vi "Edit Control File.vi"(0 "Control File Path":path, 5 "Measurement Name":string, 9 "Version":string, 11 "error in (no error)":errorcluster) -> (15 "error out":errorcluster)   [LabVIEW 2021, in "Packager Helpers.lvlib"]
uses:
  Packager Helpers.lvlib
  controls/Config File Operations.ctl
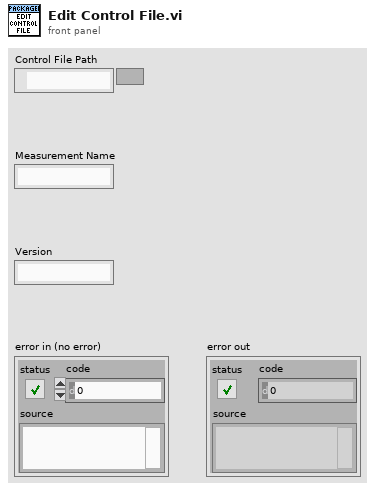
[diagram p1: front panel]
types:
  T1 = typedef "Packager Helpers.lvlib/Config File Operations.ctl" = enum16{"Read", "Write"}
  T2 = enum16{"open", "replace", "create", "open or create", "replace or create", "replace or create with confirmation"}
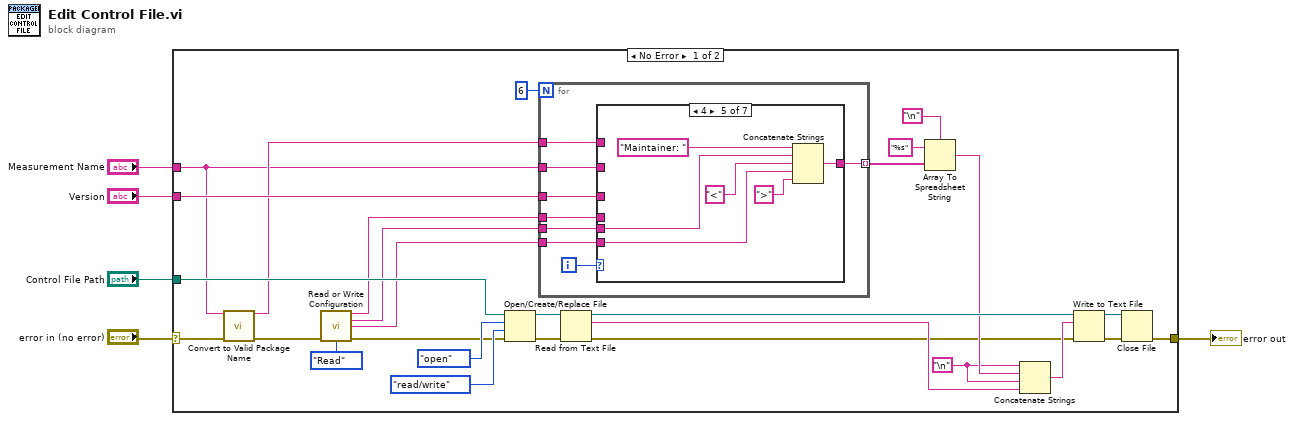
[diagram p0: block diagram]
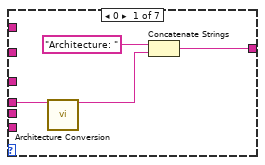
[diagram p2: hidden frame]
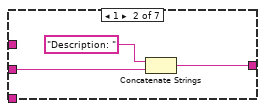
[diagram p3: hidden frame]
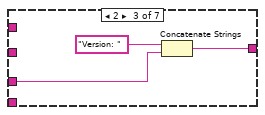
[diagram p4: hidden frame]
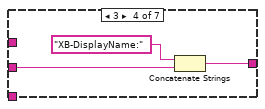
[diagram p5: hidden frame]
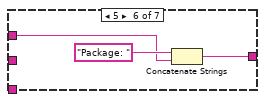
[diagram p6: hidden frame]
diagram:
  n1 = case shown="No Error" "error in (no error)" {
    selector: "error in (no error)" -> [w11 w64]
    tunnel: "Control File Path" -> [w33 _]
    tunnel: [w12 w64] -> w1
    tunnel: "Measurement Name" -> [w6 _]
    tunnel: "Version" -> [w17 _]
    frame No Error {
      w7 = "\n"
      n2 = call "Convert to Valid Package Name.vi"("Package Name"=w6, "error in (no error)"=w11) -> ("Valid Package Name"=w16:string, "error out"=w8:errorcluster)  [unwired: 12 in]
      n3 = call "Read or Write Configuration.vi"("error in (no error)"=w8, "Operation"=Config_File_Operations."Read") -> ("Architecture Out"=w20:string, "Maintainer Out"=w19:string, "Email Out"=w18:string, "error out"=w10:errorcluster)  [unwired: 10 in]
      n4 = Open/Create/Replace File(file path (use dialog)=w33, error in=w10, operation (0:open)=T2."open", access (0:read/write)=enum16{"read/write", "read-only", "write-only"}."read/write") -> (refnum out=w26:refnum<file>, error out=w9:errorcluster)  [unwired: 2 in, 1 out]
      n5 = for {
        N: 6 -> [_]
        tunnel: [w34] -> w30 mode=indexing
        tunnel: w20 -> [w40]
        tunnel: w6 -> [w39]
        tunnel: w17 -> [w38]
        tunnel: w19 -> [w37]
        tunnel: w18 -> [w36]
        tunnel: w16 -> [w35]
        i -> [w41]
        n6 = case shown="4" w41 {
          tunnel: w40 -> [w44 _ _ _ _ _ _]
          tunnel: w39 -> [_ w48 _ w53 _ _ _]
          tunnel: w38 -> [_ _ w50 _ _ _ _]
          tunnel: w37 -> [_ _ _ _ w57 _ _]
          tunnel: w36 -> [_ _ _ _ w58 _ _]
          tunnel: w35 -> [_ _ _ _ _ w62 _]
          tunnel: [w42 w46 w49 w52 w55 w61 _] -> w34
          frame 0 {
            n7 = call "Architecture Conversion.vi"("Arch In"=w44) -> ("Arch Out"=w43:string)  [unwired: 14 in]
            n8 = Concatenate Strings("Architecture: " ("regular expression"), w43) -> (w42:string)
          }
          frame 1 {
            n9 = Concatenate Strings("Description: " ("regular expression"), w48) -> (w46:string)
          }
          frame 2 {
            n10 = Concatenate Strings("Version: " ("regular expression"), w50) -> (w49:string)
          }
          frame 3 {
            n11 = Concatenate Strings("XB-DisplayName:" ("regular expression"), w53) -> (w52:string)
          }
          frame 4 {
            n12 = Concatenate Strings("Maintainer: " ("regular expression"), w57, "<" ("string"), w58, ">" ("string")) -> (w55:string)
          }
          frame 5 {
            n13 = Concatenate Strings("Package: " ("regular expression"), w62) -> (w61:string)
          }
          frame Default {
          }
        }
      }
      n14 = Read from Text File(file (use dialog)=w26, error in=w9) -> (refnum out=w25:refnum<file>, text=w22:string, error out=w14:errorcluster)  [unwired: 2 in, 1 out]
      n15 = Array To Spreadsheet String(delimiter (Tab)="\n", array=w30, 3:"%s" ("format string")) -> (spreadsheet string=w24:string)
      n16 = Concatenate Strings(w7, w24, w7, w22) -> (w23:string)
      n17 = Write to Text File(file (use dialog)=w25, text=w23, error in=w14) -> (refnum out=w27:refnum<file>, error out=w13:errorcluster)  [unwired: 1 in, 1 out]
      n18 = Close File(refnum=w27, error in=w13) -> (error out=w12:errorcluster)  [unwired: 1 out]
    }
    frame Error {
    }
  }
  "error out" <- w1
